vi "Statistic TestA.vi"(8 "This Array":u64[](array[numeric])) -> (0 "Map matching":map{string, i32}(c390), 3 "Matching array":u64[](array[numeric]), 11 "Data":i32[][](array[numeric]))   [LabVIEW 2023]
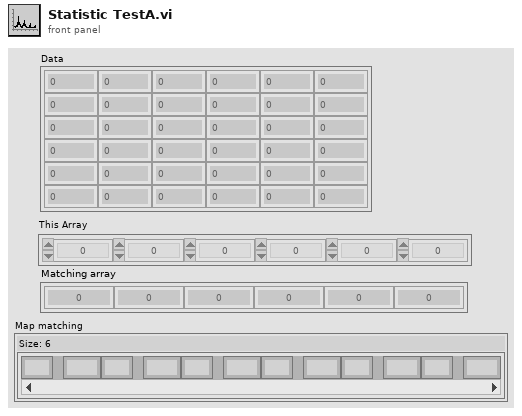
[diagram p1: front panel]
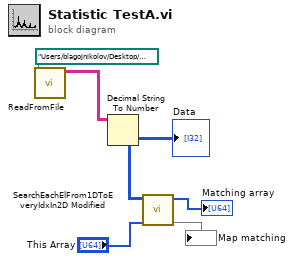
[diagram p0: block diagram]
diagram:
  n1 = call "ReadFromFile.vi"("file path (use dialog)"=path "/Users/blagojnikolov/Desktop/@tmp/test.txt" ("file path (dialog if empty)")) -> ("Array"=w6:string[][])  [unwired: 7 in, 3 out]
  n2 = Decimal String To Number(string=w6) -> (number=w4:i32[][])  [unwired: 2 in, 1 out]
  "Data" <- w4
  n3 = call "SearchEachElFrom1DToEveryIdxIn2D Modified.vi"("This Array"="This Array", "2D Target Array"=w4) -> ("Map matching"=→"Map matching":map{string, i32}, "Matching array"=→"Matching array":u64[])  [unwired: 8 in]
